vi "LV SCISDK Get Error Description.vi"(10 "handle":u64, 11 "NI Error Code":i32) -> (1 "function return":i32, 2 "handle out":u64, 3 "value":string)   [LabVIEW 2021, in "SciSDK_Labview.lvlib"]
doc: "You need this VI to call the native dll method to retrieve error description"
uses:
  SciSDK_Labview.lvlib
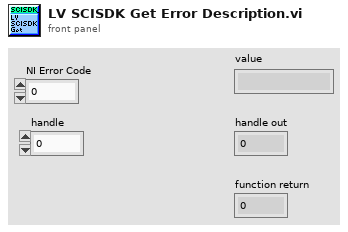
[diagram p1: front panel]
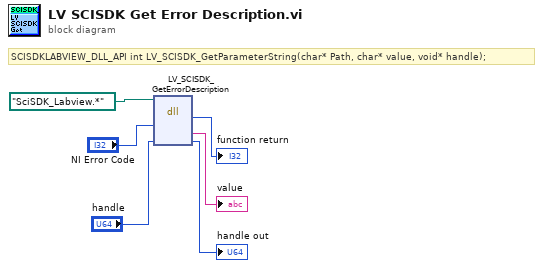
[diagram p0: block diagram]
diagram:
  # "SCISDKLABVIEW_DLL_API int LV_SCISDK_GetParameterString(char* Path, char* value, void* handle);"
  n1 = dll-call lib="C:/git/scisdk/bin/x64/Debug/SciSDK_Labview.dll" fn="LV_SCISDK_GetErrorDescription"(path in=path "SciSDK_Labview.*", "error"="NI Error Code", "handle"="handle") -> ("return type"=→"function return":i32, "value"=→"value":string, "handle"=→"handle out":u64)  [unwired: 4 in, 2 out]
